vi "Calibration File Viewer.vi"() -> ()   [LabVIEW 2020]
doc: "Visualizes the Acoustic Calibration File data for each site in 3D plot view where Amplitude, Frequency and dB SPL are represented in each axis."
uses:
  <vilib>/Math Plots/3D Math Plots/3D Surface/3D Surface XCtrl/3D Surface.xctl
  <vilib>/Math Plots/3D Math Plots/3D Surface/3D Surface Datatype/3D Surface Datatype.lvclass
  Cal File Viewer Data Cluster.ctl
  <vilib>/Math Plots/3D Math Plots/3D Plot/3D Plot Datatype/3D Plot Datatype.lvclass
  Calibration File API/Acoustic Cal Data Cluster.ctl
  <vilib>/Utility/sysdir.llb/System Directory Type.ctl
  <vilib>/Math Plots/3D Math Plots/3D Surface/3D Surface Datatype/Public/Plot Helper (Vector).vi
panel:
  out "Valid?":bool
  out "error out":errorcluster
  in  "Tab Control":T1(tab)
  out "Cal Data":refnum<class "3D Plot Datatype.lvclass">[](xcontrol)
  out "Raw Data":refnum<class "3D Plot Datatype.lvclass">[](xcontrol)
  out "Calibration Data":string[][](table)
  out "Ref Mic Cal File Data":string[][](table)=[["List Name", "40BD-FV", "", "", "", "", "", "", "", ""], ["Main Type", "40BD-FV", "", "", "", "", "", "", "", ""], ["Main Serial No", "", "", "", "", "", "", "", "", ""], ["Mic. Type", "40BD-FV", "", "", "", "", "", "", "", ""], ["Mic. Serial No", "336971", "", "", "", "", "", "", "", ""], ["PreAmp Type", "", "", "", "", "", "", "", "", ""], ["PreAmp Serial No", "", "", "", "", "", "", "", "", ""], ["", "", "", "", "", "", "", "", "", ""], ["Date & Time", "17-01-2020 09:07:50", "", "", "", "", "", "", "", ""], ["Software Version", "9.14.0.9", "", "", "", "", "", "", "", ""], ["Data File Name", "40BD-FV 336971.txt", "", "", "", "", "", "", "", ""], ["Calibration Customer ID", "", "", "", "", "", "", "", "", ""], ["Calibration ID", "", "", "", "", "", "", "", "", ""], ["Customer Item ID", "", "", "", "", "", "", "", "", ""], ["", "", "", "", "", "", "", "", "", ""], ["Operator", "HM", "", "", "", "", "", "", "", ""], ["Barometric Pressure", "1012.00", "", "", "", "", "", "", "", ""], ["Temperature", "24.00", "", "", "", "", "", "", "", ""], ["Humidity", "31.00", "", "", "", "", "", "", "", ""], ["Calibration Type", "Microphone (40xx)", "", "", "", "", "", "", "", ""], ["Adjust Coeffecient", "Disabled", "", "", "", "", "", "", "", ""], ["Coeffecient Pressure", "-0.008", "", "", "", "", "", "", "", ""], ["CoeffecientTemperature", "-0.010", "", "", "", "", "", "", "", ""], ["Coeffecient Humidity", "-0.001", "", "", "", "", "", "", "", ""], ["", "", "", "", "", "", "", "", "", ""], ["Pistonphone Name", "\"1/4\"\" Coupler\"", "", "", "", "", "", "", "", ""], ["Pistonphone Type", "42AP", "", "", "", "", "", "", "", ""], ["Pistonphone Serial Number", "68452", "", "", "", "", "", "", "", ""], ["Pistonphone Frequency [Hz]", "250.00", "", "", "", "", "", "", "", ""], ["Pistonphone Nominal Level [dB]", "114.00", "", "", "", "", "", "", "", ""], ["Pistonphone Sound Level [dB]", "114.24", "", "", "", "", "", "", "", ""], ["Pistonphone Uncertainty [dB]", "0.08", "", "", "", "", "", "", "", ""], ["Sens. Lower Limit [mV/Pa]", "1.130", "", "", "", "", "", "", "", ""], ["Sens. Nominal [mV/Pa]", "1.600", "", "", "", "", "", "", "", ""], ["Sens. Upper Limit [mV/Pa]", "2.260", "", "", "", "", "", "", "", ""], ["Sens. Volume Correction [dB]", "0.003", "", "", "", "", "", "", "", ""], ["Sens. mV/Pa", "1.372", "", "", "", "", "", "", "", ""], ["Sens. dB ref. 1V/Pa", "-57.252", "", "", "", "", "", "", "", ""], ["Sens. OK?", "OK", "", "", "", "", "", "", "", ""], ["Sens. Deviation [dB]", "-1.334", "", "", "", "", "", "", "", ""], ["Insert mV", "398.402", "", "", "", "", "", "", "", ""], ["Insert Ref mV", "431.328", "", "", "", "", "", "", "", ""], ["", "", "", "", "", "", "", "", "", ""], ["Pistonphone2 Name", "", "", "", "", "", "", "", "", ""], ["Pistonphone2 Type", "", "", "", "", "", "", "", "", ""], ["Pistonphone2 Serial Number", "", "", "", "", "", "", "", "", ""], ["Pistonphone2 Frequency [Hz]", "0.00", "", "", "", "", "", "", "", ""], ["Pistonphone2 Nominal Level [dB]", "0.00", "", "", "", "", "", "", "", ""], ["Pistonphone2 Sound Level [dB]", "0.00", "", "", "", "", "", "", "", ""], ["Pistonphone2 Uncertainty [dB]", "0.00", "", "", "", "", "", "", "", ""], ["Sens.2 Lower Limit [mV/Pa]", "1.130", "", "", "", "", "", "", "", ""], ["Sens.2 Nominal [mV/Pa]", "1.600", "", "", "", "", "", "", "", ""], ["Sens.2 Upper Limit [mV/Pa]", "2.260", "", "", "", "", "", "", "", ""], ["Sens.2 Volume Correction [dB]", "0.003", "", "", "", "", "", "", "", ""], ["Sens.2 mV/Pa", "0.000", "", "", "", "", "", "", "", ""], ["Sens.2 dB ref. 1V/Pa", "0.000", "", "", "", "", "", "", "", ""], ["Sens.2 OK?", "Fail", "", "", "", "", "", "", "", ""], ["Sens.2 Deviation [dB]", "0.000", "", "", "", "", "", "", "", ""], ["Insert2 mV", "0.000", "", "", "", "", "", "", "", ""], ["Insert2 Ref mV", "0.000", "", "", "", "", "", "", "", ""], ["", "", "", "", "", "", "", "", "", ""], ["Write TEDS OK?", "Fail", "", "", "", "", "", "", "", ""], ["TEDS memory IC", "DS2430A", "", "", "", "", "", "", "", ""], ["", "", "", "", "", "", "", "", "", ""], ["Magnitude Response OK?", "OK", "", "", "", "", "", "", "", ""], ["Normalizing Frequency [Hz]", "250.00", "", "", "", "", "", "", "", ""], ["FREQ", "Mag. Press.", "Mag. Corr.", "Other Corr.", "Ideal Mag.", "Limit+", "Limit-", "Uncertainty", "Status", "Phase"], ["250.00", "0.000", "", "", "0.000", "1.000", "-1.000", "±0.3", "OK", "-170.397"], ["280.00", "-0.002", "", "", "0.000", "1.000", "-1.000", "±0.3", "OK", "-171.558"], ["315.00", "-0.007", "", "", "0.000", "1.000", "-1.000", "±0.3", "OK", "-172.611"], ["355.00", "-0.005", "", "", "0.000", "1.000", "-1.000", "±0.3", "OK", "-173.571"], ["400.00", "-0.005", "", "", "0.000", "1.000", "-1.000", "±0.3", "OK", "-174.420"], ["450.00", "-0.008", "", "", "0.000", "1.000", "-1.000", "±0.3", "OK", "-175.205"], ["500.00", "-0.011", "", "", "0.000", "1.000", "-1.000", "±0.3", "OK", "-175.819"], ["560.00", "-0.013", "", "", "0.000", "1.000", "-1.000", "±0.3", "OK", "-176.450"], ["630.00", "-0.015", "", "", "0.000", "1.000", "-1.000", "±0.3", "OK", "-177.054"], ["710.00", "-0.016", "", "", "0.000", "1.000", "-1.000", "±0.3", "OK", "-177.621"], ["800.00", "-0.018", "", "", "0.000", "1.000", "-1.000", "±0.3", "OK", "-178.134"], ["900.00", "-0.020", "", "", "0.000", "1.000", "-1.000", "±0.3", "OK", "-178.633"], ["1000.00", "-0.021", "", "", "0.000", "1.000", "-1.000", "±0.3", "OK", "-179.062"], ["1120.00", "-0.021", "", "", "0.000", "1.000", "-1.000", "±0.3", "OK", "-179.508"], ["1250.00", "-0.022", "", "", "0.000", "1.000", "-1.000", "±0.3", "OK", "-179.909"], ["1400.00", "-0.023", "", "", "0.000", "1.000", "-1.000", "±0.3", "OK", "-180.329"], ["1600.00", "-0.025", "", "", "0.000", "1.000", "-1.000", "±0.3", "OK", "-180.849"], ["1800.00", "-0.025", "", "", "0.000", "1.000", "-1.000", "±0.3", "OK", "-181.260"], ["2000.00", "-0.017", "", "", "0.000", "1.000", "-1.000", "±0.3", "OK", "-181.741"], ["2240.00", "-0.018", "", "", "0.000", "1.000", "-1.000", "±0.3", "OK", "-182.233"], ["2500.00", "-0.016", "", "", "0.000", "1.000", "-1.000", "±0.3", "OK", "-182.723"], ["2800.00", "-0.012", "", "", "0.000", "1.000", "-1.000", "±0.3", "OK", "-183.273"], ["3150.00", "-0.009", "", "", "0.000", "1.000", "-1.000", "±0.3", "OK", "-183.889"], ["3550.00", "-0.006", "", "", "0.000", "1.000", "-1.000", "±0.3", "OK", "-184.559"], ["4000.00", "0.001", "", "", "0.000", "1.000", "-1.000", "±0.3", "OK", "-185.297"], ["4500.00", "0.009", "", "", "0.000", "1.000", "-1.000", "±0.3", "OK", "-186.103"], ["5000.00", "0.020", "", "", "0.000", "1.000", "-1.000", "±0.3", "OK", "-186.941"], ["5600.00", "0.031", "", "", "0.000", "1.000", "-1.000", "±0.3", "OK", "-187.892"], ["6300.00", "0.058", "", "", "0.000", "1.000", "-1.000", "±0.3", "OK", "-189.080"], ["7100.00", "0.076", "", "", "0.000", "1.000", "-1.000", "±0.3", "OK", "-190.285"], ["8000.00", "0.075", "", "", "0.000", "1.000", "-1.000", "±0.3", "OK", "-191.814"], ["9000.00", "0.113", "", "", "0.000", "1.000", "-1.000", "±0.3", "OK", "-193.446"], ["10000.00", "0.156", "", "", "0.000", "1.000", "-1.000", "±0.3", "OK", "-195.029"], ["11200.00", "0.194", "", "", "0.000", "1.000", "-1.000", "±0.3", "OK", "-197.182"], ["12500.00", "0.224", "", "", "0.000", "1.000", "-1.000", "±0.3", "OK", "-199.352"], ["14000.00", "0.273", "", "", "0.000", "1.000", "-1.000", "±0.3", "OK", "-202.076"], ["16000.00", "0.325", "", "", "0.000", "1.000", "-1.000", "±0.3", "OK", "-205.782"], ["18000.00", "0.356", "", "", "0.000", "1.000", "-1.000", "±0.3", "OK", "-209.740"], ["20000.00", "0.369", "", "", "0.000", "1.000", "-1.000", "±0.3", "OK", "-213.741"], ["22400.00", "0.339", "", "", "0.000", "1.000", "-1.000", "±0.3", "OK", "-218.744"], ["25000.00", "0.240", "", "", "0.000", "1.000", "-1.000", "±0.3", "OK", "-224.277"], ["28000.00", "-0.064", "", "", "0.000", "2.000", "-2.000", "±0.3", "OK", "-230.616"], ["31500.00", "-0.402", "", "", "0.000", "2.000", "-2.000", "±0.3", "OK", "-236.501"], ["35500.00", "-0.812", "", "", "0.000", "2.000", "-2.000", "±0.3", "OK", "-242.428"], ["40000.00", "-1.154", "", "", "0.000", "2.000", "-2.000", "±0.3", "OK", "-247.924"], ["45000.00", "-1.407", "", "", "0.000", "2.000", "-2.000", "±0.3", "OK", "-251.495"], ["50000.00", "-1.126", "", "", "0.000", "2.000", "-2.000", "±0.3", "OK", "-255.424"], ["56000.00", "-0.041", "", "", "0.000", "2.000", "-2.000", "±0.3", "OK", "-264.527"], ["63000.00", "0.803", "", "", "0.000", "2.000", "-2.000", "±0.3", "OK", "-283.913"], ["71000.00", "0.846", "", "", "0.000", "2.000", "-2.000", "±0.3", "OK", "-309.245"], ["80000.00", "-0.422", "", "", "0.000", "20.000", "-30.000", "±0.3", "OK", "-334.774"], ["90000.00", "-5.350", "", "", "0.000", "20.000", "-30.000", "±0.3", "OK", "-367.716"], ["100000.00", "-9.046", "", "", "0.000", "20.000", "-30.000", "±0.3", "OK", "-371.858"], ["", "", "", "", "", "", "", "", "", ""], ["", "", "", "", "", "", "", "", "", ""], ["Calibration Equipment", "", "", "", "", "", "", "", "", ""], ["641", "NI data-acquisition signal analyzer", "PCI-4461", "19709134", "Trescal", "DFM", "19-11-2019", "19-11-2021", "", ""], ["350", "Pistonphone", "42AP", "68452", "GRAS", "DFM", "19-08-2019", "19-08-2020", "42AP 68452", ""], ["970", "Pistonphone", "42AA", "306124", "GRAS", "DFM", "05-09-2019", "05-09-2020", "42AA 306124", ""], ["0", "Calibrator", "42AG", "279080", "GRAS", "DFM", "13-09-2018", "13-09-2019", "42AG 279080", ""], ["822", "1/2\" Microphone", "40AG", "88340", "GRAS", "DFM", "04-03-2019", "04-03-2020", "0806", ""], ["448", "1/4\" Microphone", "40BF", "320986", "GRAS", "DFM", "04-03-2019", "04-03-2020", "0807", ""], ["212", "Druck Barometer", "DPI 141", "14100876", "Trescal", "DTI", "18-12-2017", "18-12-2019", "22-503944", ""], ["213", "Testo Temp./Humidity probe", "0636 9735", "20180377/811", "Trescal", "DTI", "19-06-2019", "19-06-2021", "523760", ""], ["209", "Agilent Waveform Generator", "33220A", "44010793", "Trescal", "DFM", "19-11-2019", "19-11-2021", "22-530956", ""], ["243", "Agilent Multimeter", "34401A", "MY45005703", "Trescal", "DFM", "05-11-2019", "05-11-2021", "22-530251", ""], ["", "", "", "", "", "", "", "", "", ""], ["", "", "", "", "", "", "", "", "", ""], ["Comment 1", "", "", "", "", "", "", "", "", ""], ["Comment 2", "", "", "", "", "", "", "", "", ""], ["Comment 3", "", "", "", "", "", "", "", "", ""], ["Additional Remarks", "", "", "", "", "", "", "", "", ""], ["", "", "", "", "", "", "", "", "", ""]]
  in  "Select":bool
  out "Selected File":string="Show file name here"
  in  "Site":i32(ring)
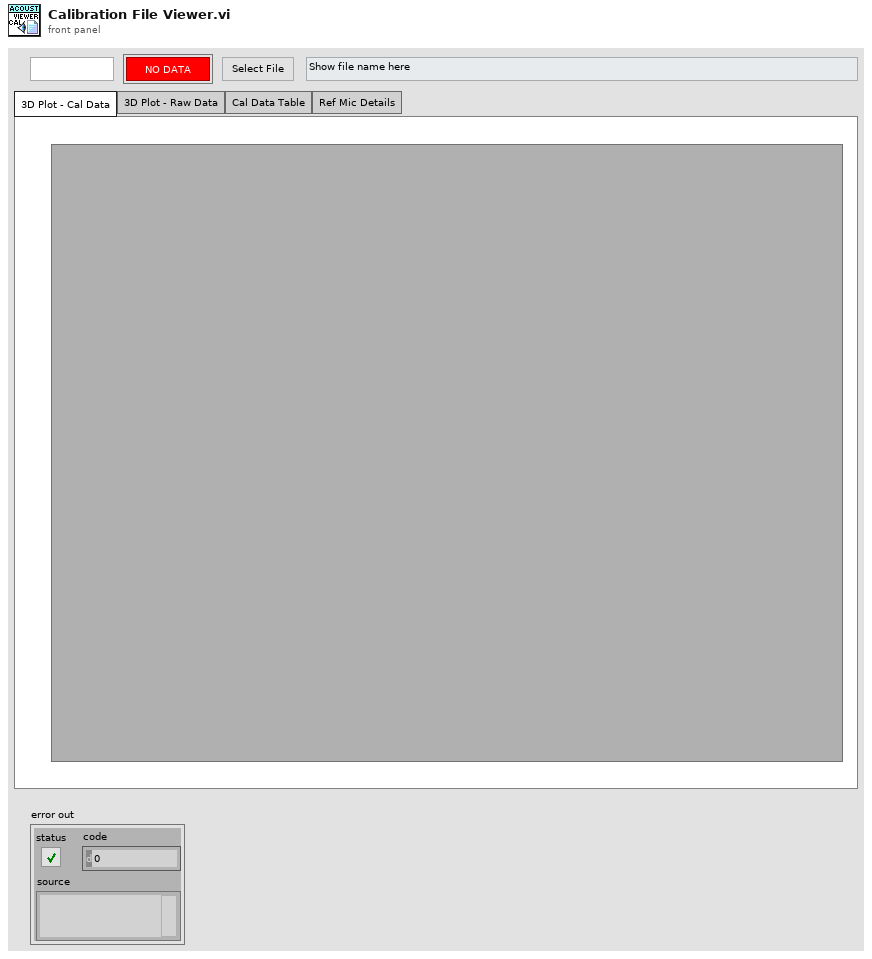
[diagram p1: front panel]
types:
  T1 = enum32{"3D Plot - Cal Data", "3D Plot - Raw Data", "Cal Data Table", "Ref Mic Details"}
  T2 = typedef "System Directory Type.ctl" = i32
  T3 = typedef "Cal File Viewer Data Cluster.ctl" = cluster{"Site":i32, "UI Selected File":string, "Cal File Path":path, "UI Calibration Data":string[][], "UI Cal Data 3D Plot":refnum<class "3D Plot Datatype.lvclass">[], "Cal File Pattern":string, "Expected Cal Location":path, "Frequency Axis":dbl[], "SPL Axis":dbl[], "Speaker Vp":dbl[][], "Cal Path Valid?":bool, "Ref Mic Cal File Data":string[][], "UI Raw Data 3D Plot":refnum<class "3D Plot Datatype.lvclass">[], "Tab":enum32{"3D Plot - Cal Data", "3D Plot - Raw Data", "Cal Data Table", "Ref Mic Details"}, "Cal File Data":T4[]}
  T4 = typedef "Acoustic Cal Data Cluster.ctl" = cluster{"Site Number":i32, "Serial Number":u32, "Ref Mic Sensitivity":dbl, "SPL Axis":dbl[], "Frequency Axis":dbl[], "Speaker Vp":dbl[][], "Ref Mic Cal File Data":string[][], "Speaker Vp Axis":dbl[], "SPL Measurements":dbl[][]}
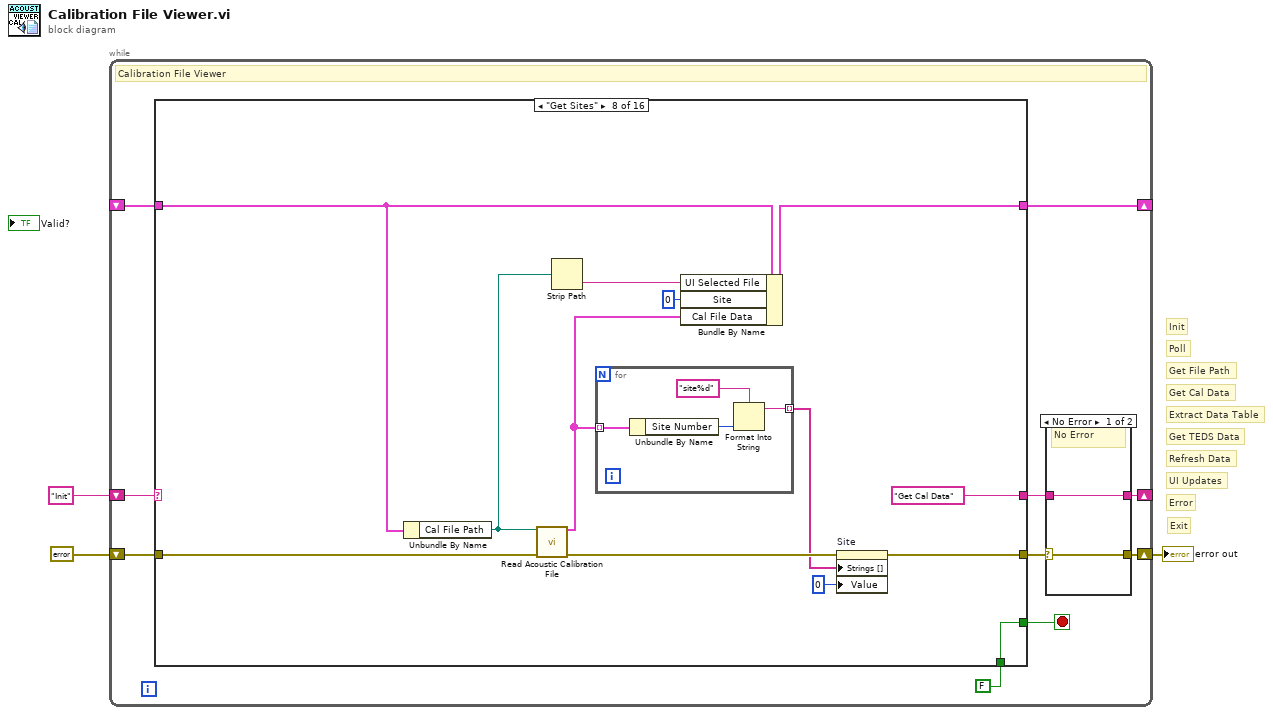
[diagram p0: block diagram]
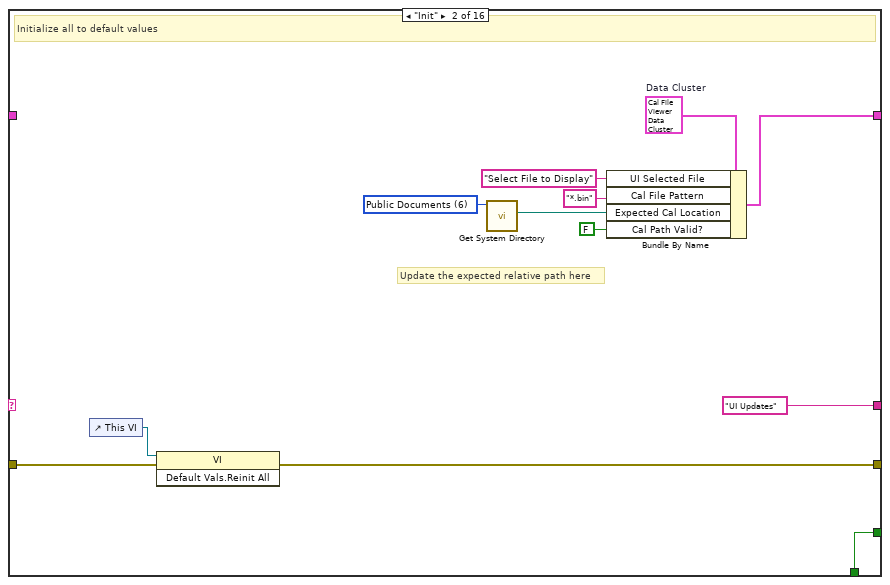
[diagram p3: hidden frame]
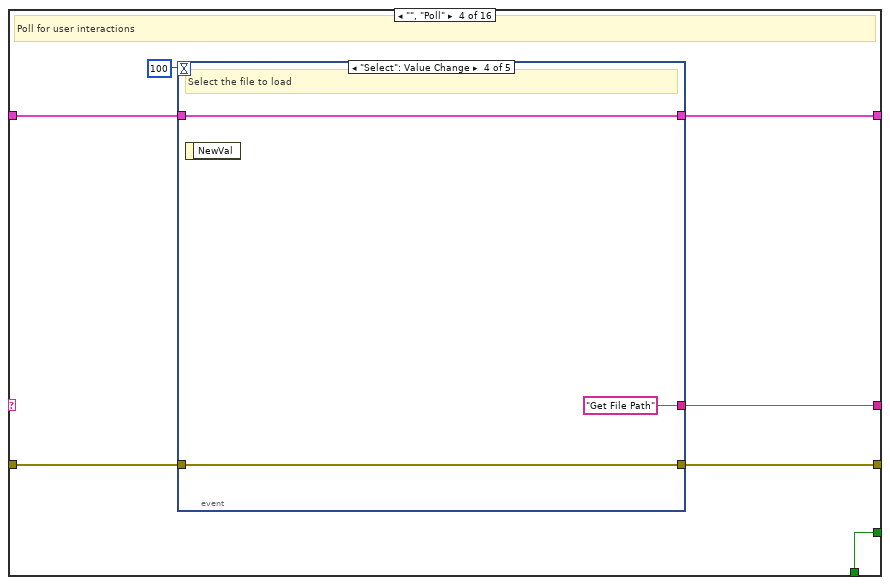
[diagram p5: hidden frame]
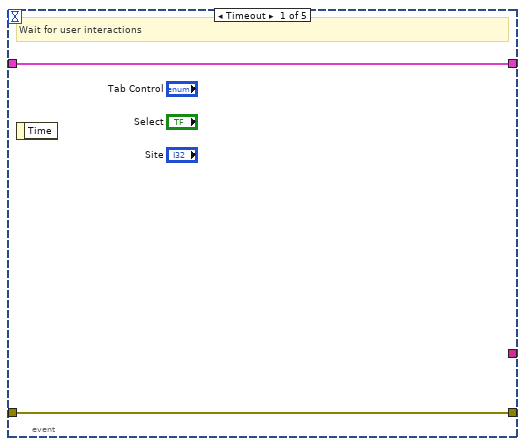
[diagram p6: hidden frame]
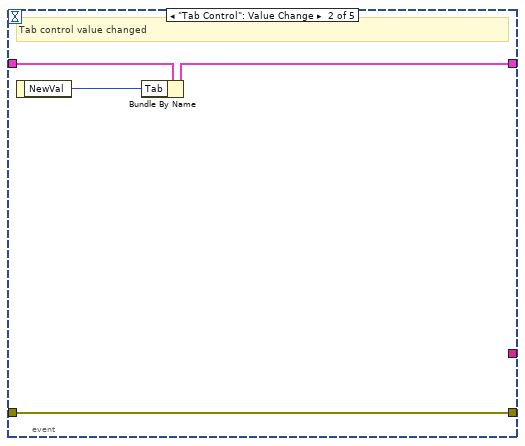
[diagram p7: hidden frame]
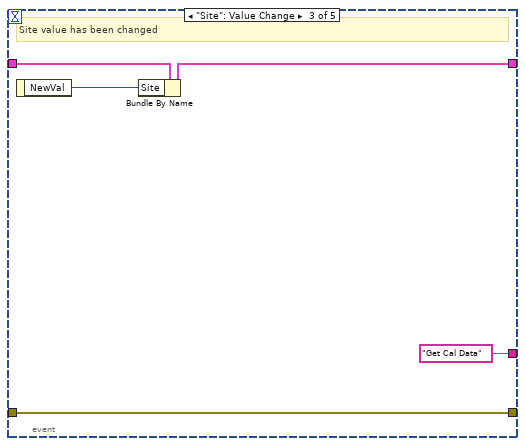
[diagram p8: hidden frame]
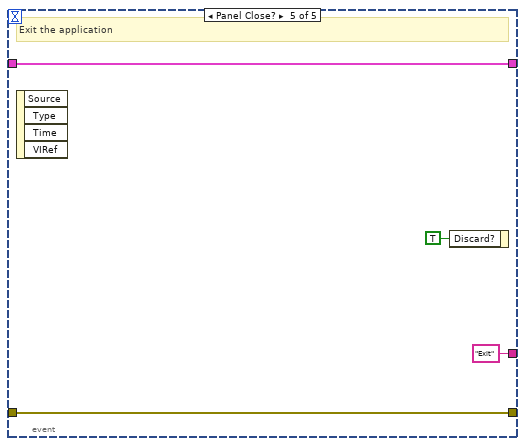
[diagram p9: hidden frame]
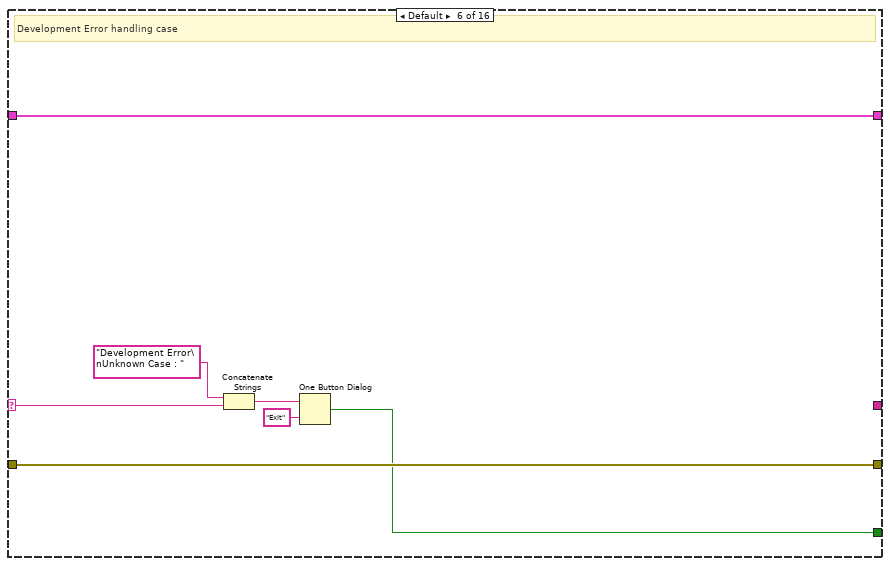
[diagram p11: hidden frame]
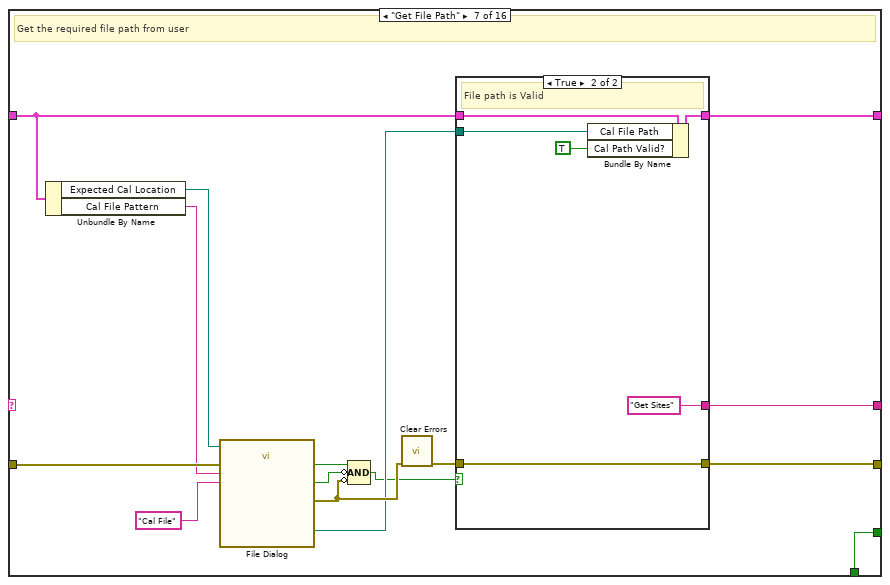
[diagram p12: hidden frame]
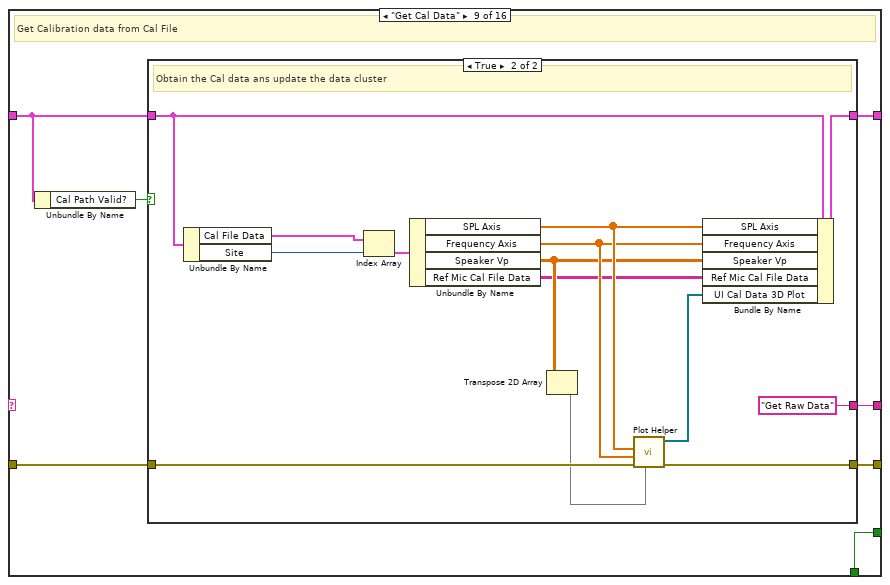
[diagram p14: hidden frame]
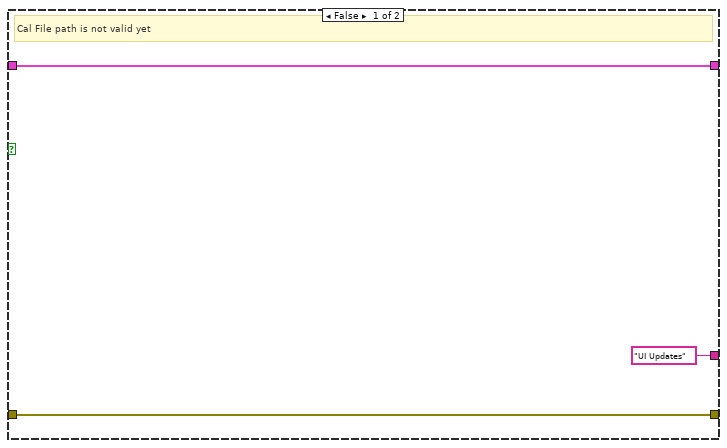
[diagram p15: hidden frame]
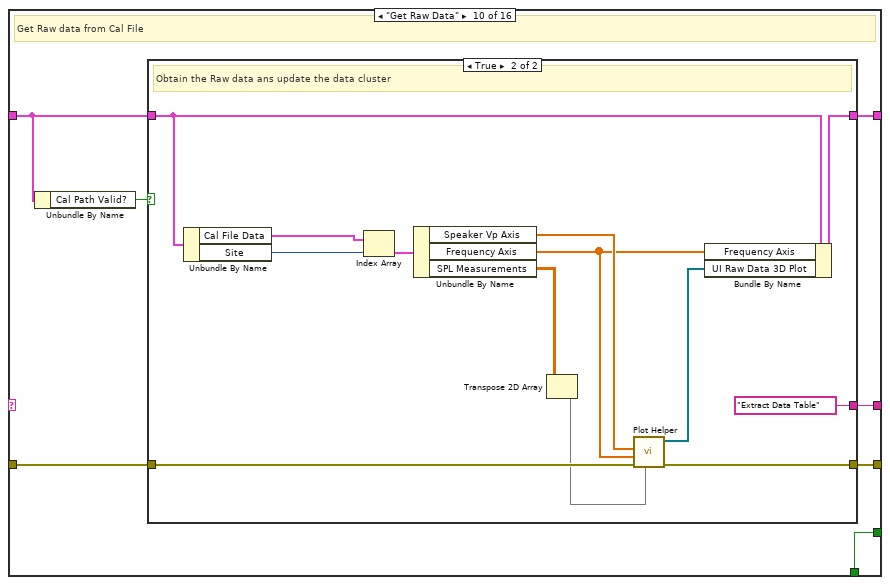
[diagram p16: hidden frame]
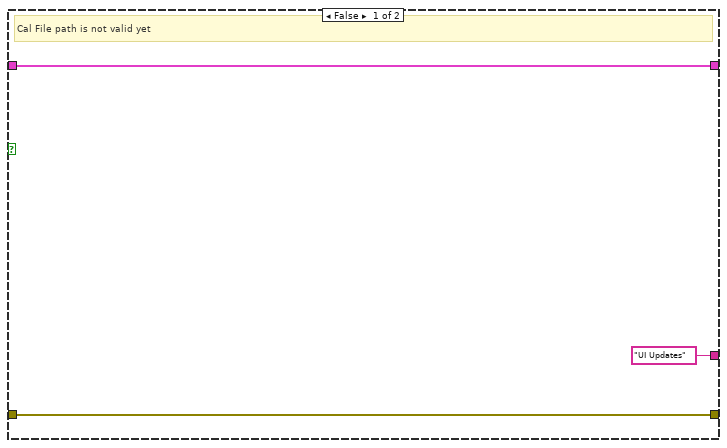
[diagram p17: hidden frame]
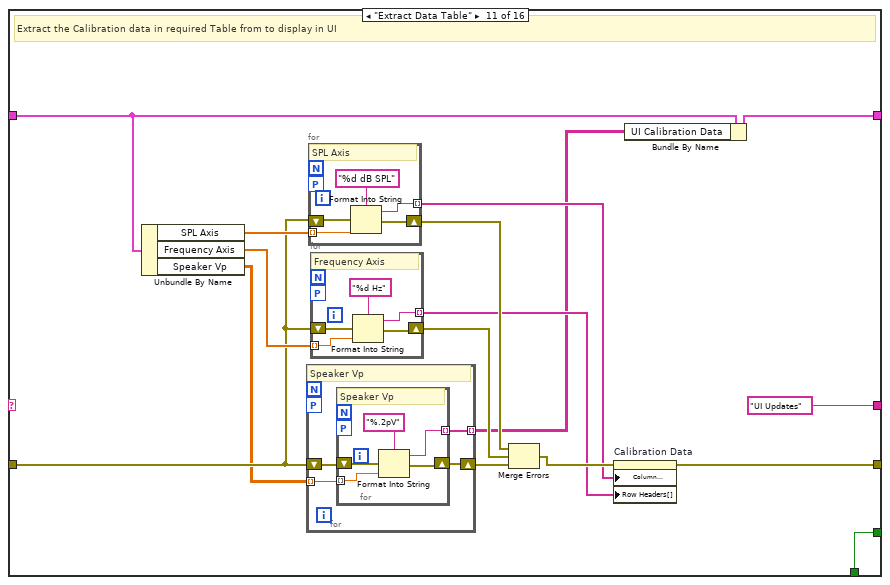
[diagram p18: hidden frame]
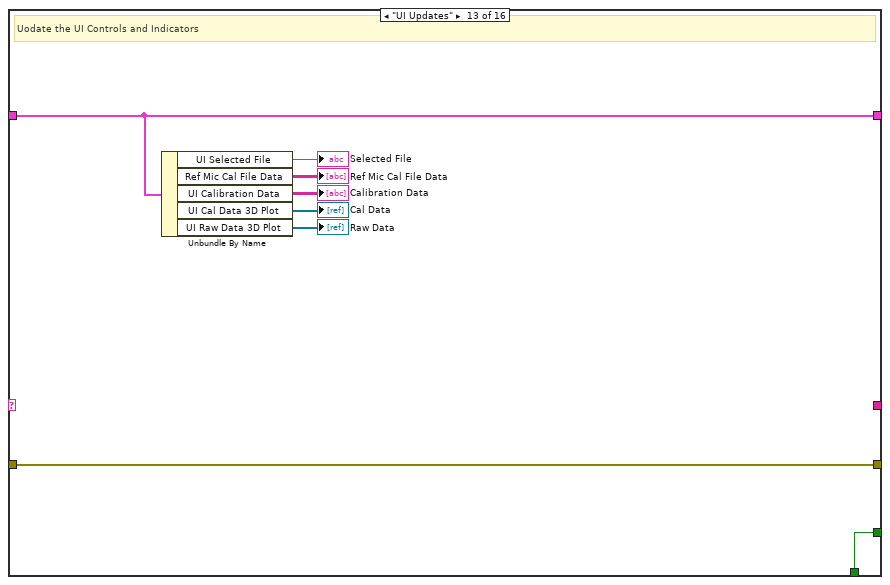
[diagram p20: hidden frame]
diagram:
  # "Exit"
  # "Error"
  # "UI Updates"
  # "Refresh Data"
  # "Get TEDS Data"
  # "Extract Data Table"
  # "Get Cal Data"
  # "Get File Path"
  # "Poll"
  # "Init"
  n1 = while {
    shift-right: [w6] -> w3
    shift-left: errorcluster {"status"=FALSE, "code"=0, "source"=""} ("error IO") -> [w13]
    shift-right: [w9] -> _
    shift-left: _ -> [w8]
    shift-right: [w5] -> _
    shift-left: "Init" -> [w10]
    stop <- w12 stop-if-true
    # "Calibration File Viewer"
    n2 = case shown="\"Get Sites\"" w10 {
      selector: w10 -> [_ _ _ _ _ w64 _ _ _ _ _ _ _ _ _ _]
      tunnel: w13 -> [w16 w25 w31 w37 w59 w66 w80 w100 w111 w135 w165 w191 w199 w202 w207 w218]
      tunnel: [w16 w24 w31 w36 w59 w66 w77 w95 w112 w136 w159 w191 w199 w202 w206 w217] -> w7
      tunnel: [w15 w28 w30 w38 w58 w60 w81 w102 w113 w137 w169 w190 w198 w201 w203 w215] -> w12
      tunnel: FALSE -> [w15 w28 w30 w38 w58 _ w81 w102 w113 w137 w169 w190 w198 w201 _ _]
      tunnel: [w14 w23 w29 w34 w57 w65 w78 w94 w110 w134 w156 w189 w197 w200 w211 w219] -> w9
      tunnel: w8 -> [w14 _ w29 w33 w57 w65 w79 w99 w108 w132 w168 w189 w197 w200 w211 w219]
      tunnel: [_ "UI Updates" _ w32 _ _ w75 "Get Cal Data" w109 w133 "UI Updates" ("f") _ _ _ _ _] -> w4
      frame "-------INIT---------" {
        # "Splitter"
      }
      frame "Init" {
        w18 = T2 6 items=["User Home"=0, "User Desktop"=1, "User Documents"=2, "User Application Data"=3, "User Preferences"=4, "User Temporary"=5, "Public Documents"=6, "Public Application Data"=7, "Public Preferences"=8, "Public Cache"=13, "System Core Libraries"=9, "System Installed Libraries"=10, "Application Files"=11, "Boot Volume Root"=12] ("system directory type")
        w27 = T3 {"Site"=0, "UI Selected File"="", "Cal File Path"=path "", "UI Calibration Data"=[], "UI Cal Data 3D Plot"=[], "Cal File Pattern"="", "Expected Cal Location"=path "", "Frequency Axis"=[], "SPL Axis"=[], "Speaker Vp"=[], "Cal Path Valid?"=FALSE, "Ref Mic Cal File Data"=[], "UI Raw Data 3D Plot"=[], "Tab"=enum."3D Plot - Cal Data", "Cal File Data"=[]}  # Data Cluster
        # "Update the expected relative path here"
        # "Initialize all to default values"
        n3 = control-ref of="This VI"() -> (w26:refnum<vi>)
        n4 = invoke class="VI" method="Default Vals.Reinit All"(reference=w26, error in=w25) -> (error out=w24:errorcluster)  [unwired: 1 in, 2 out]
        n5 = call <vilib>:"Get System Directory.vi"("system directory type"=w18) -> ("system directory"=w17:path)  [unwired: 10 in]
        n6 = Bundle By Name(cluster=w27, "UI Selected File"="Select File to Display" ("Selected File"), "Cal File Pattern"="*.bin" ("pattern (all files)"), "Expected Cal Location"=w17, "Cal Path Valid?"=FALSE) -> (w23:T3)
      }
      frame "-------POLL--------" {
        # "Splitter"
      }
      frame "", "Poll" {
        # "Poll for user interactions"
        n7 = event shown="[3] \"Select\": Value Change" {
          selector: _ -> [_ _ _ _ _]
          dyn-events: _ -> [_ _ _ _ _]
          timeout: 100 -> [_ _ _ _ _]
          tunnel: w37 -> [w40 w44 w48 w52 w56]
          tunnel: [w40 w44 w48 w52 w56] -> w36
          tunnel: [w39 w42 w47 w51 w55] -> w34
          tunnel: w33 -> [w39 w43 w49 w51 w55]
          tunnel: [_ _ "Get Cal Data" "Get File Path" "Exit"] -> w32
          event Timeout {
            # "Wait for user interactions"
            n8 = event-data() -> ()  [unwired: 1 in, 1 out]
          }
          event "Tab Control": Value Change {
            # "Tab control value changed"
            n9 = event-data() -> ("NewVal"=w41:T1)  [unwired: 1 in]
            n10 = Bundle By Name(cluster=w43, "Tab"=w41) -> (w42:T3)
          }
          event "Site": Value Change {
            # "Site value has been changed"
            n11 = event-data() -> ("NewVal"=w46:i32)  [unwired: 1 in]
            n12 = Bundle By Name(cluster=w49, "Site"=w46) -> (w47:T3)
          }
          event "Select": Value Change {
            # "Select the file to load"
            n13 = event-data() -> ()  [unwired: 1 in, 1 out]
          }
          event Panel Close? {
            # "Exit the application"
            n14 = event-data() -> ()  [unwired: 1 in, 4 out]
            n15 = event-data("Discard?"=TRUE) -> ()  [unwired: 1 in, 1 out]
          }
        }
      }
      frame "----USER EVENT----" {
        # "Splitter"
      }
      frame Default {
        # "Development Error handling case"
        n16 = Concatenate Strings("Development Error\nUnknown Case : ", w64) -> (w62:string)
        n17 = One Button Dialog(message=w62, button name ("OK")="Exit") -> (true=w60:bool)
      }
      frame "Get File Path" {
        # "Get the required file path from user"
        n18 = Unbundle By Name(w79) -> ("Expected Cal Location"=w76:path, "Cal File Pattern"=w67:string)
        n19 = call "File Dialog"("start path"=w76, "error in"=w80, "pattern (all files)"=w67, "pattern label"="Cal File") -> ("selected path"=w70:path, "exists"=w72:bool, "cancelled"=w73:bool, "error out"=w71:errorcluster)  [unwired: 8 in]
        n20 = Compound Arithmetic op=AND(w72, invert w73, invert w71) -> (w69:bool)
        n21 = call <vilib>:"Clear Errors.vi"("error in (no error)"=w71) -> ("error out"=w68:errorcluster)  [unwired: 5 in, 1 out]
        n22 = case shown="True" w69 {
          tunnel: w70 -> [_ w84]
          tunnel: w79 -> [w82 w89]
          tunnel: [w82 w88] -> w78
          tunnel: [_ "Get Sites"] -> w75
          tunnel: w68 -> [w83 w87]
          tunnel: [w83 w87] -> w77
          frame False {
            # "File not yet selected"
          }
          frame True {
            # "File path is Valid"
            n23 = Bundle By Name(cluster=w89, "Cal File Path"=w84, "Cal Path Valid?"=TRUE) -> (w88:T3)
          }
        }
      }
      frame "Get Sites" {
        n24 = Unbundle By Name(w99) -> ("Cal File Path"=w90:path)
        n25 = call "Read Acoustic Calibration File.vi"("Cal File Path"=w90, "error in (no error)"=w100) -> ("Per Site Acoustic Cal Data"=w92:T4[], "error out"=w98:errorcluster)  [unwired: 12 in]
        n26 = Strip Path(path=w90) -> (name=w91:string)  [unwired: 1 out]
        n27 = for {
          tunnel: w92 -> [w106] mode=indexing
          tunnel: [w103] -> w97 mode=indexing
          n28 = Unbundle By Name(w106) -> ("Site Number"=w104:i32)
          n29 = Format Into String(format string="site%d", w104) -> (resulting string=w103:string)  [unwired: 2 in, 1 out]
        }
        n30 = Bundle By Name(cluster=w99, "UI Selected File"=w91, "Site"=0, "Cal File Data"=w92) -> (w94:T3)
        n31 = property on="Site" class="Ring (strict)"(error in=w98, "Strings []"=w97, "Value"=0) -> (error out=w95:errorcluster)  [unwired: 1 in, 1 out]
      }
      frame "Get Cal Data" {
        # "Get Calibration data from Cal File"
        n32 = Unbundle By Name(w108) -> ("Cal Path Valid?"=w107:bool)
        n33 = case shown="True" w107 {
          tunnel: [w116 w128] -> w112
          tunnel: w111 -> [w116 w127]
          tunnel: [w115 w126] -> w110
          tunnel: ["UI Updates" ("f") "Get Raw Data" ("f")] -> w109
          tunnel: w108 -> [w115 w121]
          frame False {
            # "Cal File path is not valid yet"
          }
          frame True {
            # "Obtain the Cal data ans update the data cluster"
            n34 = Unbundle By Name(w121) -> ("Cal File Data"=w117:T4[], "Site"=w129:i32)
            n35 = Index Array(array=w117, index=w129) -> (element=w130:T4)
            n36 = Unbundle By Name(w130) -> ("SPL Axis"=w124:dbl[], "Frequency Axis"=w123:dbl[], "Speaker Vp"=w122:dbl[][], "Ref Mic Cal File Data"=w120:string[][])
            n37 = Transpose 2D Array(2D array=w122) -> (transposed array=w118:dbl[][])
            n38 = call-poly <vilib>:"Plot Helper.vi"("z matrix"=w118, "error in (no error)"=w127, "y vector"=w123, "x vector"=w124) -> ("error out"=w128:errorcluster, "3D Plot lvclass Array out"=w119:refnum<class "3D Plot Datatype.lvclass">[])  [unwired: 2 in, 4 out]
            n39 = Bundle By Name(cluster=w121, "SPL Axis"=w124, "Frequency Axis"=w123, "Speaker Vp"=w122, "Ref Mic Cal File Data"=w120, "UI Cal Data 3D Plot"=w119) -> (w126:T3)
          }
        }
      }
      frame "Get Raw Data" {
        # "Get Raw data from Cal File"
        n40 = Unbundle By Name(w132) -> ("Cal Path Valid?"=w131:bool)
        n41 = case shown="True" w131 {
          tunnel: [w140 w152] -> w136
          tunnel: w135 -> [w140 w151]
          tunnel: [w139 w150] -> w134
          tunnel: ["UI Updates" ("f") "Extract Data Table" ("f")] -> w133
          tunnel: w132 -> [w139 w145]
          frame False {
            # "Cal File path is not valid yet"
          }
          frame True {
            # "Obtain the Raw data ans update the data cluster"
            n42 = Unbundle By Name(w145) -> ("Cal File Data"=w141:T4[], "Site"=w142:i32)
            n43 = Index Array(array=w141, index=w142) -> (element=w153:T4)
            n44 = Unbundle By Name(w153) -> ("Speaker Vp Axis"=w148:dbl[], "Frequency Axis"=w147:dbl[], "SPL Measurements"=w146:dbl[][])
            n45 = Transpose 2D Array(2D array=w146) -> (transposed array=w143:dbl[][])
            n46 = call-poly <vilib>:"Plot Helper.vi"("z matrix"=w143, "error in (no error)"=w151, "y vector"=w147, "x vector"=w148) -> ("error out"=w152:errorcluster, "3D Plot lvclass Array out"=w144:refnum<class "3D Plot Datatype.lvclass">[])  [unwired: 2 in, 4 out]
            n47 = Bundle By Name(cluster=w145, "Frequency Axis"=w147, "UI Raw Data 3D Plot"=w144) -> (w150:T3)
          }
        }
      }
      frame "Extract Data Table" {
        # "Extract the Calibration data in required Table from to display in UI"
        n48 = Unbundle By Name(w168) -> ("SPL Axis"=w167:dbl[], "Frequency Axis"=w166:dbl[], "Speaker Vp"=w164:dbl[][])
        n49 = for {
          tunnel: w164 -> [w172] mode=indexing
          tunnel: [w171] -> w155 mode=indexing
          shift-right: [w170] -> w163
          shift-left: w165 -> [w173]
          workers-P: _ -> [_]
          # "Speaker Vp"
          n50 = for {
            tunnel: w172 -> [w176] mode=indexing
            tunnel: [w174] -> w171 mode=indexing
            workers-P: _ -> [_]
            shift-right: [w175] -> w170
            shift-left: w173 -> [w177]
            # "Speaker Vp"
            n51 = Format Into String(format string="%.2pV", error in=w177, w176) -> (resulting string=w174:string, error out=w175:errorcluster)  [unwired: 1 in]
          }
        }
        n52 = for {
          tunnel: w167 -> [w186] mode=indexing
          tunnel: [w184] -> w158 mode=indexing
          workers-P: _ -> [_]
          shift-right: [w185] -> w161
          shift-left: w165 -> [w187]
          # "SPL Axis"
          n53 = Format Into String(format string="%d dB SPL", error in=w187, w186) -> (resulting string=w184:string, error out=w185:errorcluster)  [unwired: 1 in]
        }
        n54 = for {
          tunnel: w166 -> [w181] mode=indexing
          tunnel: [w179] -> w157 mode=indexing
          workers-P: _ -> [_]
          shift-right: [w180] -> w162
          shift-left: w165 -> [w182]
          # "Frequency Axis"
          n55 = Format Into String(format string="%d Hz", error in=w182, w181) -> (resulting string=w179:string, error out=w180:errorcluster)  [unwired: 1 in]
        }
        n56 = Merge Errors(w161, w162, w163) -> (w160:errorcluster)
        n57 = property on="Calibration Data" class="Tbl (strict)"(error in=w160, "Column Headers[]"=w158, "Row Headers[]"=w157) -> (error out=w159:errorcluster)  [unwired: 1 in, 1 out]
        n58 = Bundle By Name(cluster=w168, "UI Calibration Data"=w155) -> (w156:T3)
      }
      frame "-----UI UPDATE-----" {
        # "Splitter"
      }
      frame "UI Updates" {
        # "Uodate the UI Controls and Indicators"
        n59 = Unbundle By Name(w197) -> ("UI Selected File"=→"Selected File":string, "Ref Mic Cal File Data"=→"Ref Mic Cal File Data":string[][], "UI Calibration Data"=→"Calibration Data":string[][], "UI Cal Data 3D Plot"=→"Cal Data":refnum<class "3D Plot Datatype.lvclass">[], "UI Raw Data 3D Plot"=→"Raw Data":refnum<class "3D Plot Datatype.lvclass">[])
      }
      frame "---ERROR & EXIT ---" {
        # "Splitter"
      }
      frame "Error" {
        # "Error has occured in the application"
        n60 = Unbundle By Name(w207) -> ("source"=w210:string)
        n61 = Concatenate Strings("Error has occured\nError Description: ", w210) -> (w208:string)
        n62 = Two Button Dialog(message=w208, 1:"Clear and Continue" ("F button name (\"Cancel\")"), 2:"Exit App" ("T button name (\"OK\")")) -> (T button?=w203:bool)
        n63 = case shown="False" w203 {
          tunnel: w207 -> [w213 w214]
          tunnel: [w212 w214] -> w206
          frame False {
            # "Clear and continue"
            n64 = call <vilib>:"Clear Errors.vi"("error in (no error)"=w213) -> ("error out"=w212:errorcluster)  [unwired: 5 in, 1 out]
          }
          frame True {
            # "Exit Application"
          }
        }
      }
      frame "Exit" {
        # "Stop the application based on User Interactions"
        n65 = Two Button Dialog(message="Stop Application?") -> (T button?=w215:bool)  [unwired: 2 in]
        n66 = case shown="False" w215 {
          tunnel: w218 -> [w220 w222]
          tunnel: [w220 w221] -> w217
          frame False {
            # "Ignore the stop"
          }
          frame True {
            # "Stop the application"
            n67 = control-ref of="This VI"() -> (w223:refnum<vi>)
            n68 = invoke class="VI" method="Default Vals.Reinit All"(reference=w223, error in=w222) -> (error out=w221:errorcluster)  [unwired: 1 in, 2 out]
          }
        }
      }
    }
    n69 = case shown="No Error" w7 {
      selector: w7 -> [w225 w227]
      tunnel: [w225 w227] -> w6
      tunnel: [w224 "Error"] -> w5
      tunnel: w4 -> [w224 _]
      frame No Error {
        # "No Error"
      }
      frame Error {
        # "Error occured"
      }
    }
  }
  "error out" <- w3
